vi "AND.vi"(8 "y":string, 11 "x":string) -> (2 "x XOR y":string)   [LabVIEW 2013]
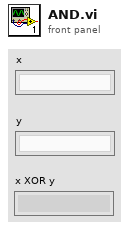
[diagram p1: front panel]
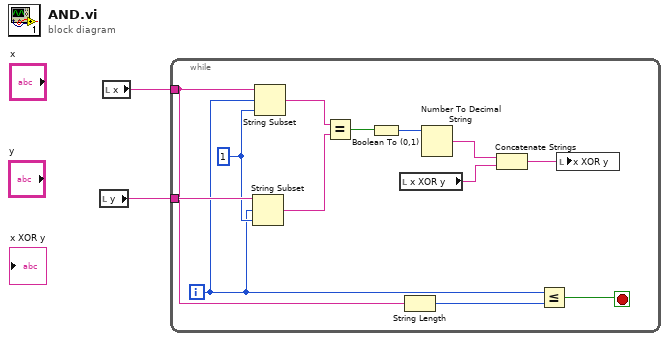
[diagram p0: block diagram]
diagram:
  n1 = local read "y"() -> (w1:string)
  n2 = local read "x"() -> (w2:string)
  n3 = while {
    tunnel: w2 -> [w4]
    tunnel: w1 -> [w15]
    i -> [w3]
    stop <- w5 stop-if-true
    w14 = 1
    n4 = String Subset(string=w15, offset (0)=w3, length (rest)=w14) -> (substring=w12:string)
    n5 = String Subset(string=w4, offset (0)=w3, length (rest)=w14) -> (substring=w13:string)
    n6 = Equal?(x=w13, y=w12) -> (x = y?=w11:bool)
    n7 = Boolean To (0,1)(Boolean=w11) -> (0, 1=w10:i16)
    n8 = local read "x XOR y"() -> (w8:string)
    n9 = String Length(string=w4) -> (length=w6:i32)
    n10 = Number To Decimal String(number=w10) -> (decimal integer string=w9:string)  [unwired: 1 in]
    n11 = Concatenate Strings(w9, w8) -> (w7:string)
    n12 = Less Or Equal?(x=w3, y=w6) -> (x <= y?=w5:bool)
    n13 = local write "x XOR y"(w7) -> ()
  }
